vi "FTIR_single.vi"() -> ()   [LabVIEW 2021]
uses:
  <vilib>/express/express analysis/Spectral/Block/exnSpectralBlock spectral measurements PSD poly.vi
  <vilib>/express/express analysis/Spectral/Block/exnSpectralBlock spectral measurements PSD DDT.vi
  <vilib>/express/express analysis/Spectral/XNode/ExpressSpectralMeasurementsBlockNode.xnode
panel:
  in  "Mirror 1 distance":dbl(slide) scale=0.05..0.25
  out "mirror 2 frequency (Hz)":dbl
  out "FFT":dynamicdata(graph)
  out "Interferogram":dynamicdata(graph)
  out "Waveform signal":dynamicdata(graph)
  out "Wavenumber k":dbl
  in  "Mirror speed":dbl(slide) scale=0.0..0.3
  out "mirror 1 frequency (Hz)":dbl
  out "Phase (deg.)":dbl
  in  "Wavelength":dbl(slide) scale=0.05..0.25
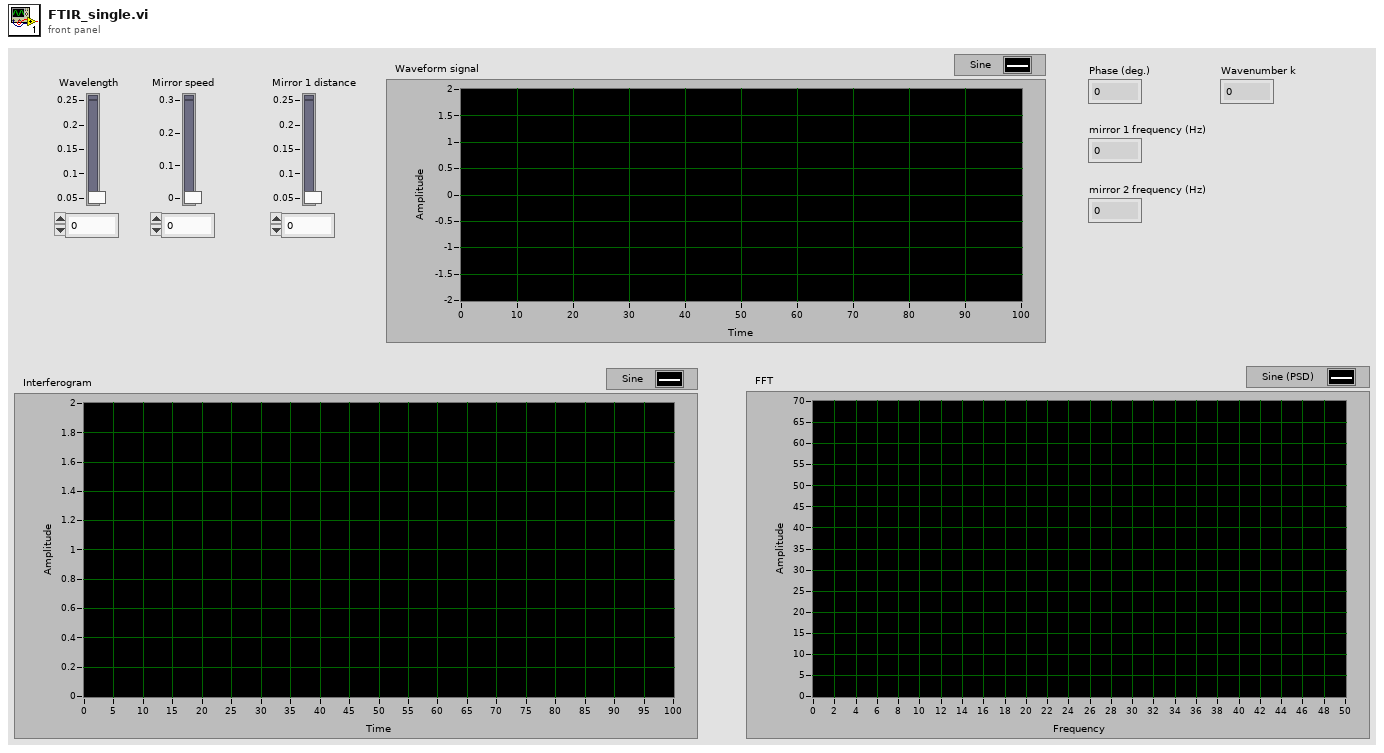
[diagram p1: front panel]
types:
  T1 = cluster{"averaging mode":u16, "weighting mode":u16, "number of averages":u32}
  T2 = cluster{"dB On (F)":bool, "unwrap phase (F)":bool, "convert to degree (F)":bool}
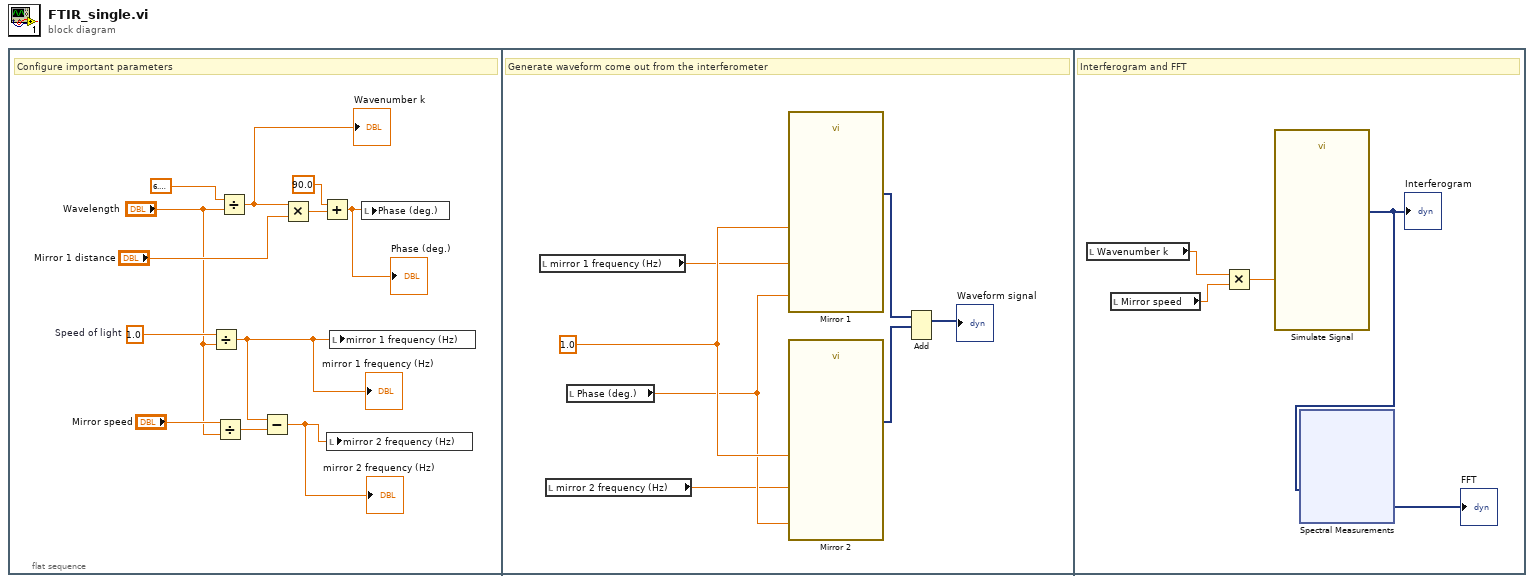
[diagram p0: block diagram]
diagram:
  n1 = flat-sequence {
    frame #0 {
      w11 = 1.0  # Speed of light
      # "Configure important parameters"
      n2 = Divide(x=w11, y="Wavelength") -> (x/y=w2:dbl)
      "mirror 1 frequency (Hz)" <- w2
      n3 = Divide(x="Mirror speed", y="Wavelength") -> (x/y=w8:dbl)
      n4 = Divide(x=6.283185307179586, y="Wavelength") -> (x/y=w4:dbl)
      "Wavenumber k" <- w4
      n5 = Subtract(x=w2, y=w8) -> (x-y=w5:dbl)
      "mirror 2 frequency (Hz)" <- w5
      n6 = Multiply(x=w4, y="Mirror 1 distance") -> (x*y=w10:dbl)
      n7 = Add(x=90.0 ("y"), y=w10) -> (x+y=w6:dbl)
      "Phase (deg.)" <- w6
      n8 = local write "mirror 2 frequency (Hz)"(w5) -> ()
      n9 = local write "mirror 1 frequency (Hz)"(w2) -> ()
      n10 = local write "Phase (deg.)"(w6) -> ()
    }
    frame #1 {
      w19 = 1.0 ("Amplitude")
      # "Generate waveform come out from the interferometer"
      n11 = local read "mirror 1 frequency (Hz)"() -> (w16:dbl)
      n12 = local read "mirror 2 frequency (Hz)"() -> (w14:dbl)
      n13 = local read "Phase (deg.)"() -> (w15:dbl)
      n14 = call "Mirror 1"("Frequency"=w16, "Amplitude"=w19, "Phase"=w15) -> ("Sine"=w18:dynamicdata)  [unwired: 11 in, 1 out]
      n15 = call "Mirror 2"("Frequency"=w14, "Amplitude"=w19, "Phase"=w15) -> ("Sine"=w17:dynamicdata)  [unwired: 11 in, 1 out]
      n16 = Add(1:w17, 2:w18) -> (0:→"Waveform signal":dynamicdata)  [unwired: 1 in, 1 out]
    }
    frame #2 {
      # "Interferogram and FFT"
      n17 = local read "Wavenumber k"() -> (w23:dbl)
      n18 = local read "Mirror speed"() -> (w22:dbl)
      n19 = Multiply(x=w23, y=w22) -> (x*y=w21:dbl)
      n20 = call "Simulate Signal"("Frequency"=w21) -> ("Sine"=w20:dynamicdata)  [unwired: 13 in, 1 out]
      "Interferogram" <- w20
      n21 = xnode "Spectral Measurements"("Signals"=w20) -> ("PSD"=→"FFT":dynamicdata)  [unwired: 1 in, 1 out]
    }
  }
